vi "Filter Predicate.vi"(1 "Element":dbl) -> (0 "Value":bool)   [LabVIEW 2020, in "Tests.lvlib"]
uses:
  Tests.lvlib
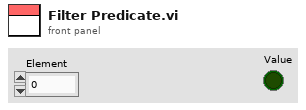
[diagram p1: front panel]
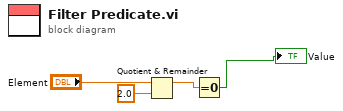
[diagram p0: block diagram]
diagram:
  n1 = Quotient & Remainder(x="Element", y=2.0) -> (x-y*floor(x/y)=w2:dbl)  [unwired: 1 out]
  n2 = Equal To 0?(x=w2) -> (x = 0?=→"Value":bool)
